vi "ExSubOMAVStrip.vi"(2 "error in (no error)":errorcluster, 3 "Camera Handle":u32) -> (0 "error out":errorcluster, 1 "Camera Handle":u32)   [LabVIEW 2010]
panel:
  # "ExSubOMAVStrip:\nThis sub-vi sets strip to single\nstrip, works best with OMA V \nor diode arrays."
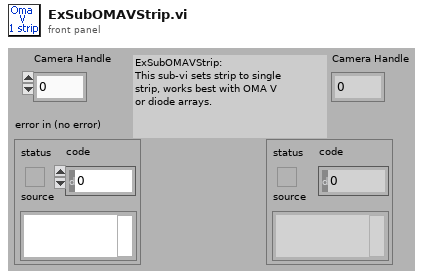
[diagram p1: front panel]
types:
  T1 = cluster{"X start":u32, "X end":u32, "X Binning/Grouping":u32, "Y start":u32, "Y end":u32, "Y Binning/Grouping":u32}
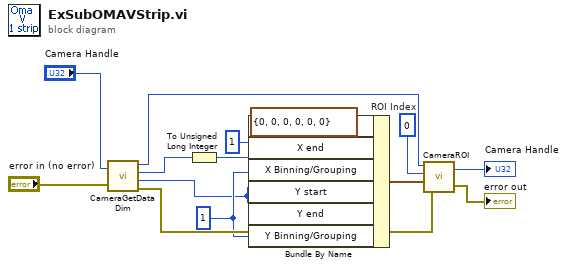
[diagram p0: block diagram]
diagram:
  w2 = u32 0  # ROI Index
  w5 = u32 1
  n1 = call <userlib>:"CameraGetDataDim.vi"("Camera Handle"="Camera Handle", "error in"="error in (no error)") -> ("Camera Handle"=w13:u32, "Xdim"=w10:u32, "Ydim"=w1:u32, "error out"=w11:errorcluster)
  n2 = To Unsigned Long Integer(number=w10) -> (unsigned 32bit integer=w6:u32)
  n3 = Bundle By Name(cluster=T1 {"X start"=0, "X end"=0, "X Binning/Grouping"=0, "Y start"=0, "Y end"=0, "Y Binning/Grouping"=0} ("ROI Params"), "X start"=u32 1, "X end"=w6, "X Binning/Grouping"=w5, "Y start"=w1, "Y end"=w1, "Y Binning/Grouping"=w5) -> (w4:T1)
  n4 = call <userlib>:"CameraROI.vi"("error in"=w11, "ROI Params"=w4, "ROI Index"=w2, "Camera Handle"=w13) -> ("error out"=→"error out":errorcluster, "Camera Handle"=→"Camera Handle":u32)
